vi "Goo01_0.vi"() -> ()   [LabVIEW 2014]
uses:
  <vilib>/myRIO/Instrument Drivers/Onboard IO/AI/vis/Read.vi
  <vilib>/myRIO/Instrument Drivers/Onboard IO/AI/vis/Smart Open.vi
  <vilib>/Utility/error.llb/Error Cluster From Error Code.vi
  <vilib>/myRIO/Common/Instrument Driver Framework/myRIO v1.0/AI/vis/myRIO v1.0 Read AI.vi
panel:
  out "원소의 인덱스":i32
  out "x-y":dbl
  # "오른쪽 수평 맞추기"
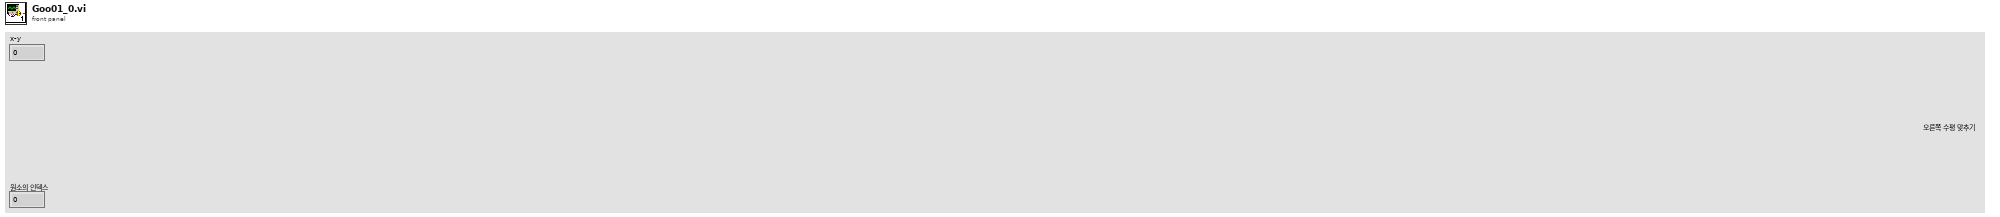
[diagram p1: front panel]
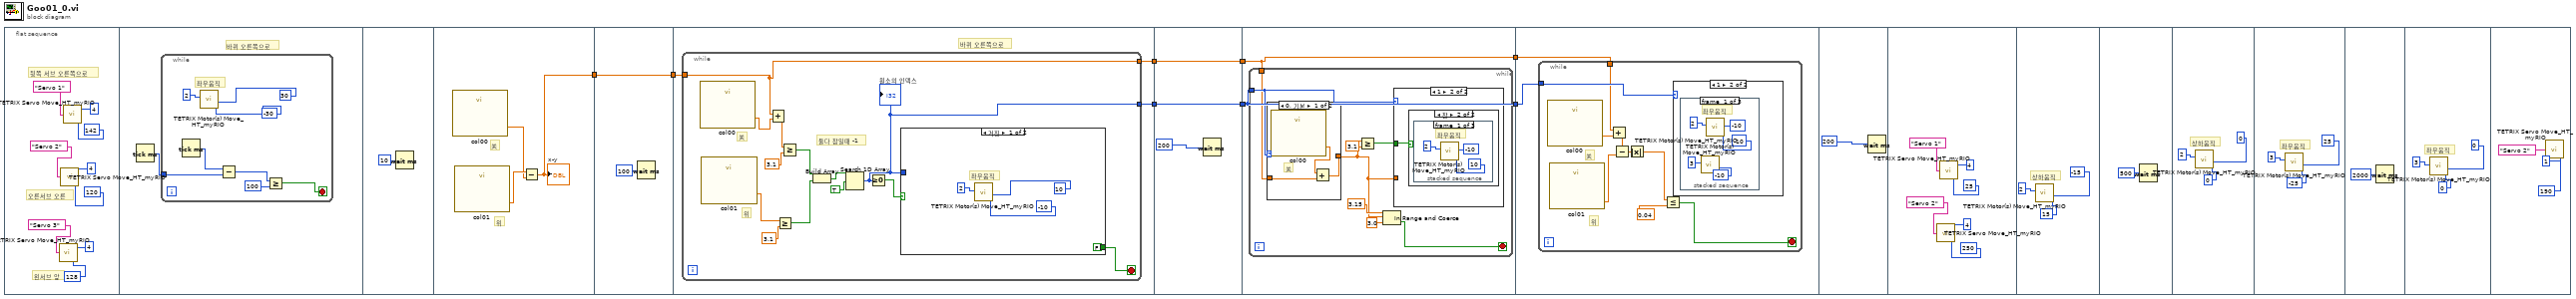
[diagram p0: block diagram]
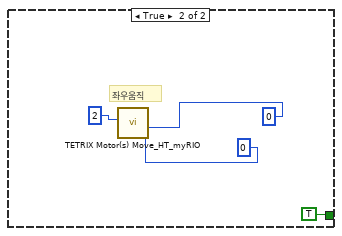
[diagram p2: hidden frame]
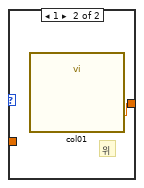
[diagram p3: hidden frame]
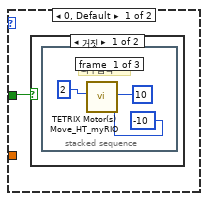
[diagram p4: hidden frame]
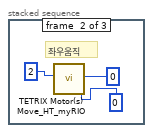
[diagram p5: hidden frame]
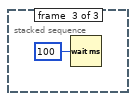
[diagram p6: hidden frame]
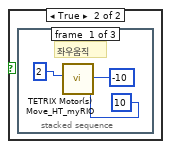
[diagram p7: hidden frame]
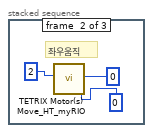
[diagram p8: hidden frame]
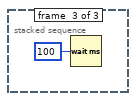
[diagram p9: hidden frame]
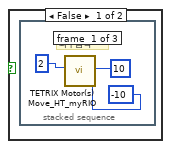
[diagram p10: hidden frame]
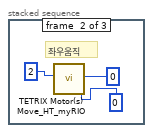
[diagram p11: hidden frame]
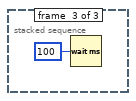
[diagram p12: hidden frame]
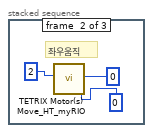
[diagram p13: hidden frame]
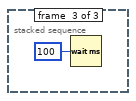
[diagram p14: hidden frame]
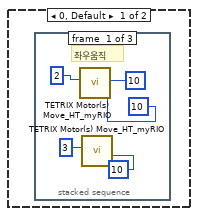
[diagram p15: hidden frame]
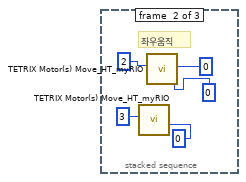
[diagram p16: hidden frame]
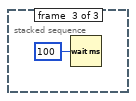
[diagram p17: hidden frame]
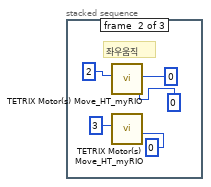
[diagram p18: hidden frame]
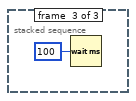
[diagram p19: hidden frame]
diagram:
  n1 = flat-sequence {
    tunnel: [w28] -> w8
    tunnel: w8 -> [w32]
    tunnel: [w32] -> w7
    tunnel: [w35] -> w6
    tunnel: w7 -> [w34]
    tunnel: [w33] -> w5
    tunnel: [w58] -> w4
    tunnel: w6 -> [w58]
    tunnel: [w57] -> w3
    tunnel: w5 -> [w57]
    tunnel: w4 -> [w61]
    tunnel: [w61] -> w2
    tunnel: w3 -> [w60]
    tunnel: [w60] -> w1
    tunnel: w2 -> [w105]
    tunnel: w1 -> [w104]
    frame #0 {
      # "왼서브 앞"
      # "오른서브 오른"
      # "뒷쪽 서브 오른쪽으로"
      n2 = call <vilib>:"TETRIX Servo Move_HT_myRIO.vi"("Servo Position (0 - 255)"=u8 128, "Controller Daisy Chain Position (1 - 4)"=u8 4, "Select Servo"="Servo 3") -> ()  [unwired: 2 in, 1 out]
      n3 = call <vilib>:"TETRIX Servo Move_HT_myRIO.vi"("Servo Position (0 - 255)"=u8 120, "Controller Daisy Chain Position (1 - 4)"=u8 4, "Select Servo"="Servo 2") -> ()  [unwired: 2 in, 1 out]
      n4 = call <vilib>:"TETRIX Servo Move_HT_myRIO.vi"("Servo Position (0 - 255)"=u8 142, "Controller Daisy Chain Position (1 - 4)"=u8 4, "Select Servo"="Servo 1") -> ()  [unwired: 2 in, 1 out]
    }
    frame #1 {
      # "바퀴 오른쪽으로"
      n5 = Tick Count (ms)() -> (millisecond timer value=w18:u32)
      n6 = while {
        tunnel: w18 -> [w22]
        stop <- w19 stop-if-true
        # "좌우움직"
        n7 = Tick Count (ms)() -> (millisecond timer value=w23:u32)
        n8 = call <vilib>:"TETRIX Motor(s) Move_HT_myRIO.vi"("Motor 2 Power (-100 to 100)\n0 = Stop/Brake\n-128 = Stop/Coast"=i8 -30 ("Motor 2 Power (-100 to 100)\n0 = Stop/Brake\n-128 = Stop/Coast"), "Motor 1 Power (-100 to 100)\n0 = Stop/Brake\n-128 = Stop/Coast"=i8 30 ("Motor 1 Power (-100 to 100)\n0 = Stop/Brake\n-128 = Stop/Coast"), "Controller Daisy Chain Position: 1 - 4"=u8 2) -> ()  [unwired: 6 in, 1 out]
        n9 = Subtract(x=w23, y=w22) -> (x-y=w21:u32)
        n10 = Greater Or Equal?(x=w21, y=u32 100) -> (x >= y?=w19:bool)
      }
    }
    frame #2 {
      n11 = Wait (ms)(milliseconds to wait=u32 10 ("대기 시간(ms)")) -> ()  [unwired: 1 out]
    }
    frame #3 {
      # "위"
      # "关"
      n12 = call "col00.vi"() -> ("Col00 (B/AI0 (Pin 3))"=w29:dbl)  [unwired: 26 in, 1 out]
      n13 = call "col01.vi"() -> ("Col01 (B/AI1 (Pin 5))"=w30:dbl)  [unwired: 26 in, 1 out]
      n14 = Subtract(x=w30, y=w29) -> (x-y=w28:dbl)
      "x-y" <- w28
    }
    frame #4 {
      n15 = Wait (ms)(milliseconds to wait=u32 100 ("대기 시간(ms)")) -> ()  [unwired: 1 out]
    }
    frame #5 {
      # "바퀴 오른쪽으로"
      n16 = while {
        tunnel: [w39] -> w35
        tunnel: w34 -> [w36]
        tunnel: [w36] -> w33
        stop <- w41 stop-if-true
        # "위"
        # "关"
        # "둘다 참일때 -1"
        n17 = call "col00.vi"() -> ("Col00 (B/AI0 (Pin 3))"=w38:dbl)  [unwired: 26 in, 1 out]
        n18 = call "col01.vi"() -> ("Col01 (B/AI1 (Pin 5))"=w40:dbl)  [unwired: 26 in, 1 out]
        n19 = Add(x=w36, y=w38) -> (x+y=w37:dbl)
        n20 = Greater Or Equal?(x=w40, y=3.1) -> (x >= y?=w45:bool)
        n21 = Greater Or Equal?(x=w37, y=3.1) -> (x >= y?=w44:bool)
        n22 = Build Array(w44, w45) -> (w48:bool[])
        n23 = Search 1D Array(1D array=w48, element=TRUE ("원소")) -> (index of element=w39:i32)  [unwired: 1 in]
        "원소의 인덱스" <- w39
        n24 = Greater Or Equal To 0?(x=w39) -> (x >= 0?=w46:bool)
        n25 = case shown="거짓" w46 {
          tunnel: w39 -> [_ _]
          tunnel: [FALSE TRUE] -> w41
          frame False {
            # "좌우움직"
            n26 = call <vilib>:"TETRIX Motor(s) Move_HT_myRIO.vi"("Motor 2 Power (-100 to 100)\n0 = Stop/Brake\n-128 = Stop/Coast"=i8 -10 ("Motor 2 Power (-100 to 100)\n0 = Stop/Brake\n-128 = Stop/Coast"), "Motor 1 Power (-100 to 100)\n0 = Stop/Brake\n-128 = Stop/Coast"=i8 10 ("Motor 1 Power (-100 to 100)\n0 = Stop/Brake\n-128 = Stop/Coast"), "Controller Daisy Chain Position: 1 - 4"=u8 2) -> ()  [unwired: 6 in, 1 out]
          }
          frame True {
            # "좌우움직"
            n27 = call <vilib>:"TETRIX Motor(s) Move_HT_myRIO.vi"("Motor 2 Power (-100 to 100)\n0 = Stop/Brake\n-128 = Stop/Coast"=i8 0 ("Motor 2 Power (-100 to 100)\n0 = Stop/Brake\n-128 = Stop/Coast"), "Motor 1 Power (-100 to 100)\n0 = Stop/Brake\n-128 = Stop/Coast"=i8 0 ("Motor 1 Power (-100 to 100)\n0 = Stop/Brake\n-128 = Stop/Coast"), "Controller Daisy Chain Position: 1 - 4"=u8 2) -> ()  [unwired: 6 in, 1 out]
          }
        }
      }
    }
    frame #6 {
      n28 = Wait (ms)(milliseconds to wait=u32 200 ("대기 시간(ms)")) -> ()  [unwired: 1 out]
    }
    frame #7 {
      n29 = while {
        tunnel: w61 -> [w69]
        tunnel: w60 -> [w62]
        stop <- w68 stop-if-true
        n30 = case shown="0, 기본" w69 {
          tunnel: [w70 w73] -> w63
          tunnel: w62 -> [w72 _]
          frame 0, Default {
            # "关"
            n31 = call "col00.vi"() -> ("Col00 (B/AI0 (Pin 3))"=w71:dbl)  [unwired: 26 in, 1 out]
            n32 = Add(x=w71, y=w72) -> (x+y=w70:dbl)
          }
          frame 1 {
            # "위"
            n33 = call "col01.vi"() -> ("Col01 (B/AI1 (Pin 5))"=w73:dbl)  [unwired: 26 in, 1 out]
          }
        }
        n34 = Greater Or Equal?(x=w63, y=3.1) -> (x >= y?=w64:bool)
        n35 = In Range and Coerce(upper limit=3.15 ("y"), x=w63, lower limit=3.0 ("하위 리미트")) -> (In Range?=w68:bool)  [unwired: 1 out]
        n36 = case shown="1" w69 {
          tunnel: w63 -> [_ _]
          tunnel: w64 -> [w74 w89]
          frame 0, Default {
            n37 = case shown="거짓" w74 {
              frame False {
                n38 = stacked-sequence {
                  frame #0 {
                    # "좌우움직"
                    n39 = call <vilib>:"TETRIX Motor(s) Move_HT_myRIO.vi"("Motor 2 Power (-100 to 100)\n0 = Stop/Brake\n-128 = Stop/Coast"=i8 -10 ("Motor 2 Power (-100 to 100)\n0 = Stop/Brake\n-128 = Stop/Coast"), "Motor 1 Power (-100 to 100)\n0 = Stop/Brake\n-128 = Stop/Coast"=i8 10 ("Motor 1 Power (-100 to 100)\n0 = Stop/Brake\n-128 = Stop/Coast"), "Controller Daisy Chain Position: 1 - 4"=u8 2) -> ()  [unwired: 6 in, 1 out]
                  }
                  frame #1 {
                    # "좌우움직"
                    n40 = call <vilib>:"TETRIX Motor(s) Move_HT_myRIO.vi"("Motor 2 Power (-100 to 100)\n0 = Stop/Brake\n-128 = Stop/Coast"=i8 0 ("Motor 2 Power (-100 to 100)\n0 = Stop/Brake\n-128 = Stop/Coast"), "Motor 1 Power (-100 to 100)\n0 = Stop/Brake\n-128 = Stop/Coast"=i8 0 ("Motor 1 Power (-100 to 100)\n0 = Stop/Brake\n-128 = Stop/Coast"), "Controller Daisy Chain Position: 1 - 4"=u8 2) -> ()  [unwired: 6 in, 1 out]
                  }
                  frame #2 {
                    n41 = Wait (ms)(milliseconds to wait=u32 100 ("대기 시간(ms)")) -> ()  [unwired: 1 out]
                  }
                }
              }
              frame True {
                n42 = stacked-sequence {
                  frame #0 {
                    # "좌우움직"
                    n43 = call <vilib>:"TETRIX Motor(s) Move_HT_myRIO.vi"("Motor 2 Power (-100 to 100)\n0 = Stop/Brake\n-128 = Stop/Coast"=i8 10 ("Motor 2 Power (-100 to 100)\n0 = Stop/Brake\n-128 = Stop/Coast"), "Motor 1 Power (-100 to 100)\n0 = Stop/Brake\n-128 = Stop/Coast"=i8 -10 ("Motor 1 Power (-100 to 100)\n0 = Stop/Brake\n-128 = Stop/Coast"), "Controller Daisy Chain Position: 1 - 4"=u8 2) -> ()  [unwired: 6 in, 1 out]
                  }
                  frame #1 {
                    # "좌우움직"
                    n44 = call <vilib>:"TETRIX Motor(s) Move_HT_myRIO.vi"("Motor 2 Power (-100 to 100)\n0 = Stop/Brake\n-128 = Stop/Coast"=i8 0 ("Motor 2 Power (-100 to 100)\n0 = Stop/Brake\n-128 = Stop/Coast"), "Motor 1 Power (-100 to 100)\n0 = Stop/Brake\n-128 = Stop/Coast"=i8 0 ("Motor 1 Power (-100 to 100)\n0 = Stop/Brake\n-128 = Stop/Coast"), "Controller Daisy Chain Position: 1 - 4"=u8 2) -> ()  [unwired: 6 in, 1 out]
                  }
                  frame #2 {
                    n45 = Wait (ms)(milliseconds to wait=u32 100 ("대기 시간(ms)")) -> ()  [unwired: 1 out]
                  }
                }
              }
            }
          }
          frame 1 {
            n46 = case shown="참" w89 {
              frame False {
                n47 = stacked-sequence {
                  frame #0 {
                    # "좌우움직"
                    n48 = call <vilib>:"TETRIX Motor(s) Move_HT_myRIO.vi"("Motor 2 Power (-100 to 100)\n0 = Stop/Brake\n-128 = Stop/Coast"=i8 -10 ("Motor 2 Power (-100 to 100)\n0 = Stop/Brake\n-128 = Stop/Coast"), "Motor 1 Power (-100 to 100)\n0 = Stop/Brake\n-128 = Stop/Coast"=i8 10 ("Motor 1 Power (-100 to 100)\n0 = Stop/Brake\n-128 = Stop/Coast"), "Controller Daisy Chain Position: 1 - 4"=u8 2) -> ()  [unwired: 6 in, 1 out]
                  }
                  frame #1 {
                    # "좌우움직"
                    n49 = call <vilib>:"TETRIX Motor(s) Move_HT_myRIO.vi"("Motor 2 Power (-100 to 100)\n0 = Stop/Brake\n-128 = Stop/Coast"=i8 0 ("Motor 2 Power (-100 to 100)\n0 = Stop/Brake\n-128 = Stop/Coast"), "Motor 1 Power (-100 to 100)\n0 = Stop/Brake\n-128 = Stop/Coast"=i8 0 ("Motor 1 Power (-100 to 100)\n0 = Stop/Brake\n-128 = Stop/Coast"), "Controller Daisy Chain Position: 1 - 4"=u8 2) -> ()  [unwired: 6 in, 1 out]
                  }
                  frame #2 {
                    n50 = Wait (ms)(milliseconds to wait=u32 100 ("대기 시간(ms)")) -> ()  [unwired: 1 out]
                  }
                }
              }
              frame True {
                n51 = stacked-sequence {
                  frame #0 {
                    # "좌우움직"
                    n52 = call <vilib>:"TETRIX Motor(s) Move_HT_myRIO.vi"("Motor 2 Power (-100 to 100)\n0 = Stop/Brake\n-128 = Stop/Coast"=i8 10 ("Motor 2 Power (-100 to 100)\n0 = Stop/Brake\n-128 = Stop/Coast"), "Motor 1 Power (-100 to 100)\n0 = Stop/Brake\n-128 = Stop/Coast"=i8 -10 ("Motor 1 Power (-100 to 100)\n0 = Stop/Brake\n-128 = Stop/Coast"), "Controller Daisy Chain Position: 1 - 4"=u8 2) -> ()  [unwired: 6 in, 1 out]
                  }
                  frame #1 {
                    # "좌우움직"
                    n53 = call <vilib>:"TETRIX Motor(s) Move_HT_myRIO.vi"("Motor 2 Power (-100 to 100)\n0 = Stop/Brake\n-128 = Stop/Coast"=i8 0 ("Motor 2 Power (-100 to 100)\n0 = Stop/Brake\n-128 = Stop/Coast"), "Motor 1 Power (-100 to 100)\n0 = Stop/Brake\n-128 = Stop/Coast"=i8 0 ("Motor 1 Power (-100 to 100)\n0 = Stop/Brake\n-128 = Stop/Coast"), "Controller Daisy Chain Position: 1 - 4"=u8 2) -> ()  [unwired: 6 in, 1 out]
                  }
                  frame #2 {
                    n54 = Wait (ms)(milliseconds to wait=u32 100 ("대기 시간(ms)")) -> ()  [unwired: 1 out]
                  }
                }
              }
            }
          }
        }
      }
    }
    frame #8 {
      n55 = while {
        tunnel: w105 -> [w114]
        tunnel: w104 -> [w108]
        stop <- w110 stop-if-true
        # "위"
        # "关"
        n56 = call "col00.vi"() -> ("Col00 (B/AI0 (Pin 3))"=w107:dbl)  [unwired: 26 in, 1 out]
        n57 = call "col01.vi"() -> ("Col01 (B/AI1 (Pin 5))"=w113:dbl)  [unwired: 26 in, 1 out]
        n58 = Add(x=w108, y=w107) -> (x+y=w106:dbl)
        n59 = Subtract(x=w106, y=w113) -> (x-y=w112:dbl)
        n60 = Absolute Value(x=w112) -> (abs(x)=w111:dbl)
        n61 = Less Or Equal?(x=w111, y=0.04) -> (x <= y?=w110:bool)
        n62 = case shown="1" w114 {
          frame 0, Default {
            n63 = stacked-sequence {
              frame #0 {
                # "좌우움직"
                n64 = call <vilib>:"TETRIX Motor(s) Move_HT_myRIO.vi"("Motor 2 Power (-100 to 100)\n0 = Stop/Brake\n-128 = Stop/Coast"=i8 10 ("Motor 2 Power (-100 to 100)\n0 = Stop/Brake\n-128 = Stop/Coast"), "Motor 1 Power (-100 to 100)\n0 = Stop/Brake\n-128 = Stop/Coast"=i8 10 ("Motor 1 Power (-100 to 100)\n0 = Stop/Brake\n-128 = Stop/Coast"), "Controller Daisy Chain Position: 1 - 4"=u8 2) -> ()  [unwired: 6 in, 1 out]
                n65 = call <vilib>:"TETRIX Motor(s) Move_HT_myRIO.vi"("Motor 1 Power (-100 to 100)\n0 = Stop/Brake\n-128 = Stop/Coast"=i8 10 ("Motor 1 Power (-100 to 100)\n0 = Stop/Brake\n-128 = Stop/Coast"), "Controller Daisy Chain Position: 1 - 4"=u8 3) -> ()  [unwired: 7 in, 1 out]
              }
              frame #1 {
                # "좌우움직"
                n66 = call <vilib>:"TETRIX Motor(s) Move_HT_myRIO.vi"("Motor 1 Power (-100 to 100)\n0 = Stop/Brake\n-128 = Stop/Coast"=i8 0 ("Motor 1 Power (-100 to 100)\n0 = Stop/Brake\n-128 = Stop/Coast"), "Controller Daisy Chain Position: 1 - 4"=u8 3) -> ()  [unwired: 7 in, 1 out]
                n67 = call <vilib>:"TETRIX Motor(s) Move_HT_myRIO.vi"("Motor 2 Power (-100 to 100)\n0 = Stop/Brake\n-128 = Stop/Coast"=i8 0 ("Motor 2 Power (-100 to 100)\n0 = Stop/Brake\n-128 = Stop/Coast"), "Motor 1 Power (-100 to 100)\n0 = Stop/Brake\n-128 = Stop/Coast"=i8 0 ("Motor 1 Power (-100 to 100)\n0 = Stop/Brake\n-128 = Stop/Coast"), "Controller Daisy Chain Position: 1 - 4"=u8 2) -> ()  [unwired: 6 in, 1 out]
              }
              frame #2 {
                n68 = Wait (ms)(milliseconds to wait=u32 100 ("대기 시간(ms)")) -> ()  [unwired: 1 out]
              }
            }
          }
          frame 1 {
            n69 = stacked-sequence {
              frame #0 {
                # "좌우움직"
                n70 = call <vilib>:"TETRIX Motor(s) Move_HT_myRIO.vi"("Motor 1 Power (-100 to 100)\n0 = Stop/Brake\n-128 = Stop/Coast"=i8 -10 ("Motor 1 Power (-100 to 100)\n0 = Stop/Brake\n-128 = Stop/Coast"), "Controller Daisy Chain Position: 1 - 4"=u8 3) -> ()  [unwired: 7 in, 1 out]
                n71 = call <vilib>:"TETRIX Motor(s) Move_HT_myRIO.vi"("Motor 2 Power (-100 to 100)\n0 = Stop/Brake\n-128 = Stop/Coast"=i8 -10 ("Motor 2 Power (-100 to 100)\n0 = Stop/Brake\n-128 = Stop/Coast"), "Motor 1 Power (-100 to 100)\n0 = Stop/Brake\n-128 = Stop/Coast"=i8 -10 ("Motor 1 Power (-100 to 100)\n0 = Stop/Brake\n-128 = Stop/Coast"), "Controller Daisy Chain Position: 1 - 4"=u8 2) -> ()  [unwired: 6 in, 1 out]
              }
              frame #1 {
                # "좌우움직"
                n72 = call <vilib>:"TETRIX Motor(s) Move_HT_myRIO.vi"("Motor 2 Power (-100 to 100)\n0 = Stop/Brake\n-128 = Stop/Coast"=i8 0 ("Motor 2 Power (-100 to 100)\n0 = Stop/Brake\n-128 = Stop/Coast"), "Motor 1 Power (-100 to 100)\n0 = Stop/Brake\n-128 = Stop/Coast"=i8 0 ("Motor 1 Power (-100 to 100)\n0 = Stop/Brake\n-128 = Stop/Coast"), "Controller Daisy Chain Position: 1 - 4"=u8 2) -> ()  [unwired: 6 in, 1 out]
                n73 = call <vilib>:"TETRIX Motor(s) Move_HT_myRIO.vi"("Motor 1 Power (-100 to 100)\n0 = Stop/Brake\n-128 = Stop/Coast"=i8 0 ("Motor 1 Power (-100 to 100)\n0 = Stop/Brake\n-128 = Stop/Coast"), "Controller Daisy Chain Position: 1 - 4"=u8 3) -> ()  [unwired: 7 in, 1 out]
              }
              frame #2 {
                n74 = Wait (ms)(milliseconds to wait=u32 100 ("대기 시간(ms)")) -> ()  [unwired: 1 out]
              }
            }
          }
        }
      }
    }
    frame #9 {
      n75 = Wait (ms)(milliseconds to wait=u32 200 ("대기 시간(ms)")) -> ()  [unwired: 1 out]
    }
    frame #10 {
      n76 = call <vilib>:"TETRIX Servo Move_HT_myRIO.vi"("Servo Position (0 - 255)"=u8 250, "Controller Daisy Chain Position (1 - 4)"=u8 4, "Select Servo"="Servo 2") -> ()  [unwired: 2 in, 1 out]
      n77 = call <vilib>:"TETRIX Servo Move_HT_myRIO.vi"("Servo Position (0 - 255)"=u8 25, "Controller Daisy Chain Position (1 - 4)"=u8 4, "Select Servo"="Servo 1") -> ()  [unwired: 2 in, 1 out]
    }
    frame #11 {
      # "상하움직"
      n78 = call <vilib>:"TETRIX Motor(s) Move_HT_myRIO.vi"("Motor 2 Power (-100 to 100)\n0 = Stop/Brake\n-128 = Stop/Coast"=i8 15 ("Motor 2 Power (-100 to 100)\n0 = Stop/Brake\n-128 = Stop/Coast"), "Motor 1 Power (-100 to 100)\n0 = Stop/Brake\n-128 = Stop/Coast"=i8 -15 ("Motor 1 Power (-100 to 100)\n0 = Stop/Brake\n-128 = Stop/Coast"), "Controller Daisy Chain Position: 1 - 4"=u8 2) -> ()  [unwired: 6 in, 1 out]
    }
    frame #12 {
      n79 = Wait (ms)(milliseconds to wait=u32 500 ("대기 시간(ms)")) -> ()  [unwired: 1 out]
    }
    frame #13 {
      # "상하움직"
      n80 = call <vilib>:"TETRIX Motor(s) Move_HT_myRIO.vi"("Motor 2 Power (-100 to 100)\n0 = Stop/Brake\n-128 = Stop/Coast"=i8 0 ("Motor 2 Power (-100 to 100)\n0 = Stop/Brake\n-128 = Stop/Coast"), "Motor 1 Power (-100 to 100)\n0 = Stop/Brake\n-128 = Stop/Coast"=i8 0 ("Motor 1 Power (-100 to 100)\n0 = Stop/Brake\n-128 = Stop/Coast"), "Controller Daisy Chain Position: 1 - 4"=u8 2) -> ()  [unwired: 6 in, 1 out]
    }
    frame #14 {
      # "좌우움직"
      n81 = call <vilib>:"TETRIX Motor(s) Move_HT_myRIO.vi"("Motor 2 Power (-100 to 100)\n0 = Stop/Brake\n-128 = Stop/Coast"=i8 -25 ("Motor 2 Power (-100 to 100)\n0 = Stop/Brake\n-128 = Stop/Coast"), "Motor 1 Power (-100 to 100)\n0 = Stop/Brake\n-128 = Stop/Coast"=i8 25 ("Motor 1 Power (-100 to 100)\n0 = Stop/Brake\n-128 = Stop/Coast"), "Controller Daisy Chain Position: 1 - 4"=u8 3) -> ()  [unwired: 6 in, 1 out]
    }
    frame #15 {
      n82 = Wait (ms)(milliseconds to wait=u32 2000 ("대기 시간(ms)")) -> ()  [unwired: 1 out]
    }
    frame #16 {
      # "좌우움직"
      n83 = call <vilib>:"TETRIX Motor(s) Move_HT_myRIO.vi"("Motor 2 Power (-100 to 100)\n0 = Stop/Brake\n-128 = Stop/Coast"=i8 0 ("Motor 2 Power (-100 to 100)\n0 = Stop/Brake\n-128 = Stop/Coast"), "Motor 1 Power (-100 to 100)\n0 = Stop/Brake\n-128 = Stop/Coast"=i8 0 ("Motor 1 Power (-100 to 100)\n0 = Stop/Brake\n-128 = Stop/Coast"), "Controller Daisy Chain Position: 1 - 4"=u8 3) -> ()  [unwired: 6 in, 1 out]
    }
    frame #17 {
      n84 = call <vilib>:"TETRIX Servo Move_HT_myRIO.vi"("Servo Position (0 - 255)"=u8 190, "Controller Daisy Chain Position (1 - 4)"=u8 1, "Select Servo"="Servo 2") -> ()  [unwired: 2 in, 1 out]
    }
  }
